vi "getLogicOutChannel.vi"(8 "error in (no error)":errorcluster, 11 "pHandle":u32) -> (0 "error out":errorcluster, 1 "return type":i32, 2 "polarityStr":string, 3 "outputTypeStr":string)   [LabVIEW 2011, in "sbgLabView.lvlib"]
uses:
  sbgLabView.lvlib
  sbgMatLab.dll
panel:
  out "duration":u8
  in  "channel":u8
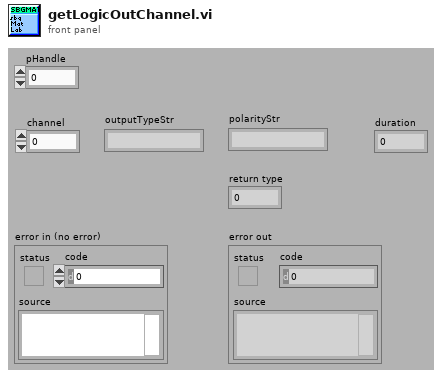
[diagram p1: front panel]
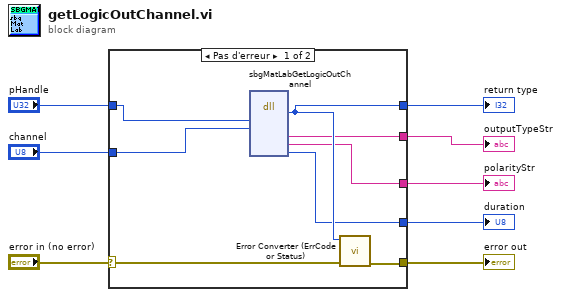
[diagram p0: block diagram]
diagram:
  n1 = case shown="Pas d'erreur" "error in (no error)" {
    selector: "error in (no error)" -> [w12 w17]
    tunnel: [w11 w17] -> w7
    tunnel: [w16 _] -> w6
    tunnel: "pHandle" -> [w15 _]
    tunnel: [w14 _] -> w4
    tunnel: [w13 _] -> w3
    tunnel: "channel" -> [w10 _]
    tunnel: [w9 _] -> w1
    frame No Error {
      n2 = dll-call lib="C:/SBG-Systems/remote/projects/software/projects/labviewExample/sbgLabView/sbgMatLab.*" fn="sbgMatLabGetLogicOutChannel" ("sbgMatLab.dll:sbgMatLabGetGpsOptions")("pHandle"=w15, "channel"=w10) -> ("type de retour"=w16:i32, "outputTypeStr"=w14:string, "polarityStr"=w13:string, "pDuration"=w9:u8)  [unwired: 8 in, 2 out]
      n3 = call "Error Converter (ErrCode or Status).vi"("error in (no error)"=w12, "error code"=w16) -> ("error out"=w11:errorcluster)  [unwired: 9 in]
    }
    frame Error {
    }
  }
  "return type" <- w6
  "outputTypeStr" <- w4
  "polarityStr" <- w3
  "error out" <- w7
  "duration" <- w1
